vi "Set Maximum Velocity.vi"(4 "error in (no error)":errorcluster, 5 "Maximum Velocity (0 units/s)":dbl min=0.0 max=2000000000.0 format="%.6g", 6 "Axis (1)":i32=1 min=1 max=3, 7 "VISA resource name":refnum<visa-resource-name>) -> (0 "error out":errorcluster, 3 "VISA resource name out":refnum<visa-resource-name>)   [LabVIEW 2018, in "Newport ESP301.lvlib"]
doc: "This command is used to set the maximum velocity value for an axis. This command remains effective even if the requested axis is member of a group. In this case an error message, \"GROUP MAXIMUM VELOCITY EXCEEDED\", is generated if the commanded value is less than group velocity. (Refer to Advanced Capabilities section for a detailed description of grouping and related commands)."
uses:
  Newport ESP301.lvlib
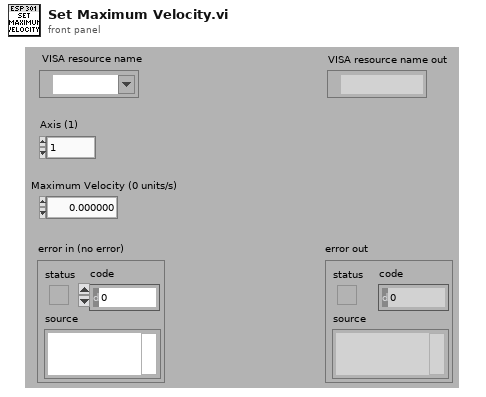
[diagram p1: front panel]
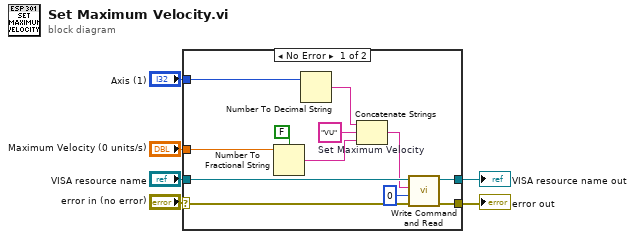
[diagram p0: block diagram]
diagram:
  n1 = case shown="No Error" "error in (no error)" {
    selector: "error in (no error)" -> [w15 w20]
    tunnel: [w17 w20] -> w6
    tunnel: "VISA resource name" -> [w18 w19]
    tunnel: [w16 w19] -> w5
    tunnel: "Axis (1)" -> [w12 _]
    tunnel: "Maximum Velocity (0 units/s)" -> [w10 _]
    frame No Error {
      w14 = "VU"  # Set Maximum Velocity
      n2 = Number To Fractional String(use system decimal point (T)=FALSE ("utiliser le séparateur décimal du système (V)"), number=w10) -> (F-format string=w9:string)  [unwired: 2 in]
      n3 = Number To Decimal String(number=w12) -> (decimal integer string=w13:string)  [unwired: 1 in]
      n4 = Concatenate Strings(w13, w14, w9) -> (w11:string)
      n5 = call "Write Command and Read.vi"("error in (no error)"=w15, "Bytes to read (100)"=u32 0, "Command"=w11, "VISA resource name"=w18) -> ("error out"=w17:errorcluster, "VISA resource name out"=w16:refnum<visa-resource-name>)  [unwired: 3 in, 1 out]
    }
    frame Error {
    }
  }
  "error out" <- w6
  "VISA resource name out" <- w5
